vi "N330X_CC_Configuration.vi"(0 "VISA resource name":refnum<visa-resource-name>, 1 "Regulation Mode (0:Current)":i32(ring) items=["Current", "Resistance", "Voltage"], 5 "Channel (1)":u32=1, 7 "Input Current Range (1 A)":dbl=1.0, 9 "Input Current (1 A)":dbl=1.0, 11 "error in (no error)":errorcluster, 12 "Current Measurement Range (1 A)":dbl=1.0) -> (15 "error out":errorcluster)   [LabVIEW 2015]
panel:
  in  "Trigger Source (2: Hold)":i32(ring)=2 items=["Bus", "External", "Hold", "Line", "Timer"]
  in  "Regulator (0:Fixed)":i32(ring) items=["Fixed", "List"]
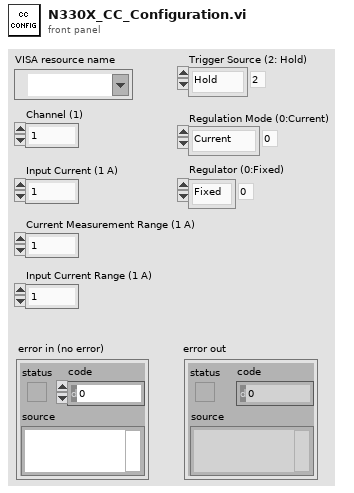
[diagram p1: front panel]
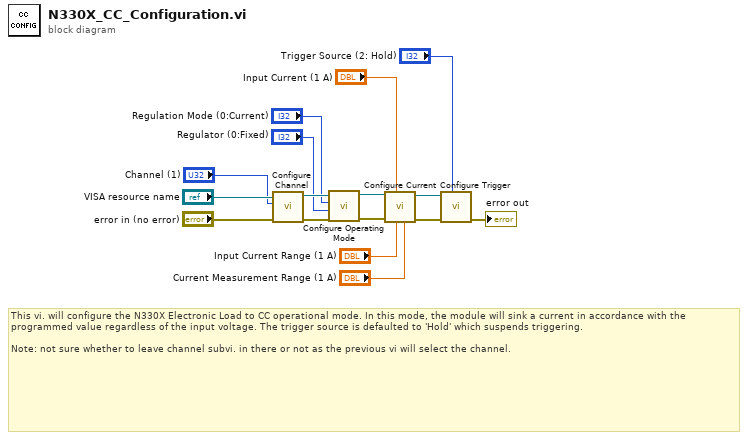
[diagram p0: block diagram]
diagram:
  # "This vi. will configure the N330X Electronic Load to CC operational mode. In this mode, the module will sink a current in accordance with the programmed value regardless of the input voltage. The trigger source is defaulted to 'Hold' which suspends triggering.  \n\nNote: not sure whether to leave channel subvi. in there or not as the previous vi will select the channel."
  n1 = call <instrlib>:"Configure Channel.vi"("error in (no error)"="error in (no error)", "Channel (1)"="Channel (1)", "VISA resource name"="VISA resource name") -> ("error out"=w7:errorcluster, "VISA resource name out"=w8:refnum<visa-resource-name>)  [unwired: 7 in]
  n2 = call <instrlib>:"Configure Operating Mode.vi"("error in (no error)"=w7, "Regulator (0:Fixed)"="Regulator (0:Fixed)", "Regulation Mode (0:Current)"="Regulation Mode (0:Current)", "VISA resource name"=w8) -> ("error out"=w5:errorcluster, "VISA resource name out"=w6:refnum<visa-resource-name>)  [unwired: 6 in]
  n3 = call <instrlib>:"Configure Current.vi"("Current Measurement Range (1 A)"="Current Measurement Range (1 A)", "Input Current Range (1 A)"="Input Current Range (1 A)", "Input Current (1 A)"="Input Current (1 A)", "error in (no error)"=w5, "VISA resource name"=w6) -> ("error out"=w16:errorcluster, "VISA resource name out"=w15:refnum<visa-resource-name>)  [unwired: 5 in]
  n4 = call <instrlib>:"Configure Trigger.vi"("Trigger Source (2: Hold)"="Trigger Source (2: Hold)", "error in (no error)"=w16, "VISA resource name"=w15) -> ("error out"=→"error out":errorcluster)  [unwired: 7 in, 1 out]
